vi "DRAM read write process.vi"(5 "debug ctr reset":bool, 6 "dram.reset":bool, 8 "dram mode":T3, 11 "DRAM resources":T1={"DRAM read data FIFO"="", "DRAM write data FIFO"="", "DRAM request FIFO"="", "DRAM U512 memo"=refnum, "DMA data loader"="custom data", "BRAM read data FIFO"="", "BRAM write data FIFO"="", "BRAM request FIFO"="", "BRAM U512 memo"=refnum}) -> (2 "DRAM debug ctr":T2, 3 "last written addr":u32)   [LabVIEW 2019, in "TX burst sequencer.lvlib"]
doc: "Handles writing and reading from DRAM.\nHas 3 interface FIFOs:\n- Write FIFO: provides data to write (addr + data)\n- Request FIFO: provides requests for data read\n- Read FIFO: takes data read from DRAM\n\nVI has 3 main states:\n- write (only write operations are executed with max throughput)\n- read (only read operations are executed with max throughput)\n- flush (empties Write and Request FIFO)"
uses:
  TX burst sequencer.lvlib
  DRAM mode.ctl
  DRAM resources.ctl
  <instrlib>/_niInstr/Memory/v1/FPGA/DRAM U512/niInstr Memory DRAM U512 v1 FPGA.lvclass
  <instrlib>/_niInstr/Memory/v1/FPGA/BRAM U512/niInstr Memory BRAM U512 v1 FPGA.lvclass
  <instrlib>/_niInstr/Memory/v1/FPGA/Memory/Public/Write Data (With Byte Enables).ctl
  <instrlib>/_niInstr/Memory/v1/FPGA/Memory/Public/Read Request.ctl
  <instrlib>/_niInstr/Memory/v1/FPGA/DRAM/Public/Timeslot Arbiter Configuration.ctl
  <vilib>/rvi/DataTransferAndStorage/Container/Common/niFpgaContainerExecOnDevCompGetState.vi
  <vilib>/rvi/Emulation/niFpgaEmulationIsFPGAContextNoSignature.vi
  <vilib>/rvi/Emulation/niFpgaSctlEmulationGetInTimedLoop.vi
  <vilib>/rvi/errors/niFpgaSetErrorForExecOnDevCompSimple.vi
  <vilib>/rvi/eio/common/nirviEmuReportErrorAndStop.vi
  <vilib>/rvi/DataTransferAndStorage/Container/Common/niFpgaContainerGetUniqueNameForEmu.vi
  <vilib>/rvi/FIFO/Fifo_Resource/nirvififoEmulationSetSize.vi
  <vilib>/rvi/FIFO/Fifo_Resource/nirviFifoEmulationQueueMgr.vi
  <instcachedir>/0/nirviFifoEmulationQueueMgr_E5CAEC123FF24DC58D834DCA3CDAA9B5.lvgen/nirviFifoEmulationQueueMgr_E5CAEC123FF24DC58D834DCA3CDAA9B5_017.vi
  <vilib>/rvi/FIFO/Fifo_Resource/nirvififoEmulationDetermineInputValidOut.vi
  <vilib>/rvi/FIFO/Fifo_Resource/nirvififoEmulationCreateLock.vi
  <vilib>/rvi/Emulation/niFpgaProcessEmulError.vi
  <vilib>/rvi/FIFO/Fifo_Resource/nirvififoEmulationObtainLock.vi
  <vilib>/rvi/FIFO/Fifo_Resource/nirvififoEmulationReleaseLock.vi
  <vilib>/rvi/occurrence/nirviWaitOnOccurrenceBase.vi
  <vilib>/rvi/errors/nirviReportUnexpectedCaseInternalError.vi
  <vilib>/rvi/errors/nirviReportUnexpectedCaseInternalError (U32).vi
  <vilib>/Utility/error.llb/Clear Errors.vi
  <vilib>/rvi/interface/RandomDataEmulation/niFpgaRandomDataHandleErrors.vi
  <instcachedir>/0/nirviFifoEmulationQueueMgr_E5CAEC123FF24DC58D834DCA3CDAA9B5.lvgen/nirviFifoEmulationQueueMgr_E5CAEC123FF24DC58D834DCA3CDAA9B5_003.vi
  <instrlib>/_niInstr/Basic Elements/v1/FPGA/Private/Count Up U32.vi
  <instcachedir>/0/nirviFifoEmulationQueueMgr_E5CAEC123FF24DC58D834DCA3CDAA9B5.lvgen/nirviFifoEmulationQueueMgr_E5CAEC123FF24DC58D834DCA3CDAA9B5_011.vi
  <vilib>/rvi/DataTransferAndStorage/Container/XNode/niFpgaContainer.xnode
  <vilib>/rvi/FIFO/Fifo_Resource/niFpgaFifoEmulationRefIn.vi
  <instrlib>/_niInstr/Memory/v1/FPGA/Memory/niInstr Memory v1 FPGA.lvclass
  <instrlib>/_niInstr/Memory/v1/FPGA/DRAM/niInstr Memory DRAM v1 FPGA.lvclass
  <instrlib>/_niInstr/Basic Elements/v1/FPGA/niInstr Basic Elements v1 FPGA.lvlib
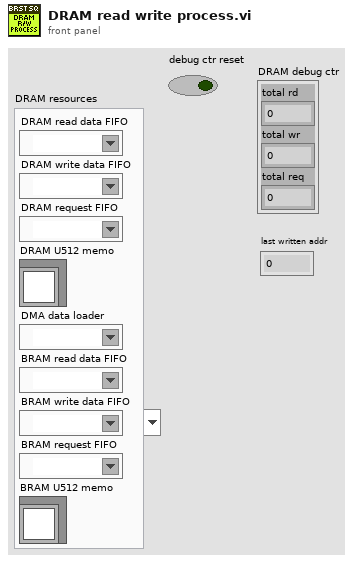
[diagram p1: front panel]
types:
  T1 = typedef "TX burst sequencer.lvlib/DRAM resources.ctl" = cluster{"DRAM read data FIFO":refnum<k21>, "DRAM write data FIFO":refnum<k21>, "DRAM request FIFO":refnum<k21>, "DRAM U512 memo":refnum<class "niInstr Memory DRAM U512 v1 FPGA.lvclass">, "DMA data loader":refnum<k21>, "BRAM read data FIFO":refnum<k21>, "BRAM write data FIFO":refnum<k21>, "BRAM request FIFO":refnum<k21>, "BRAM U512 memo":refnum<class "niInstr Memory BRAM U512 v1 FPGA.lvclass">}
  T2 = cluster{"total rd":u32, "total wr":u32, "total req":u32}
  T3 = typedef "TX burst sequencer.lvlib/DRAM mode.ctl" = enum16{"flush", "reset", "write", "read"}
  T4 = typedef "niInstr Memory v1 FPGA.lvclass/Read Request.ctl" = cluster{"address":u32, "valid":bool}
  T5 = typedef "niInstr Memory v1 FPGA.lvclass/Write Data (With Byte Enables).ctl" = cluster{"address":u32, "data":bool[], "byte enables":bool[], "valid":bool}
  T6 = typedef "niInstr Memory DRAM v1 FPGA.lvclass/Timeslot Arbiter Configuration.ctl" = cluster{"write grant time (clocks)":u16, "read grant time (clocks)":u16}
  T7 = typedef "niInstr Memory v1 FPGA.lvclass/Retrieve Data.ctl" = cluster{"data":bool[], "valid":bool}
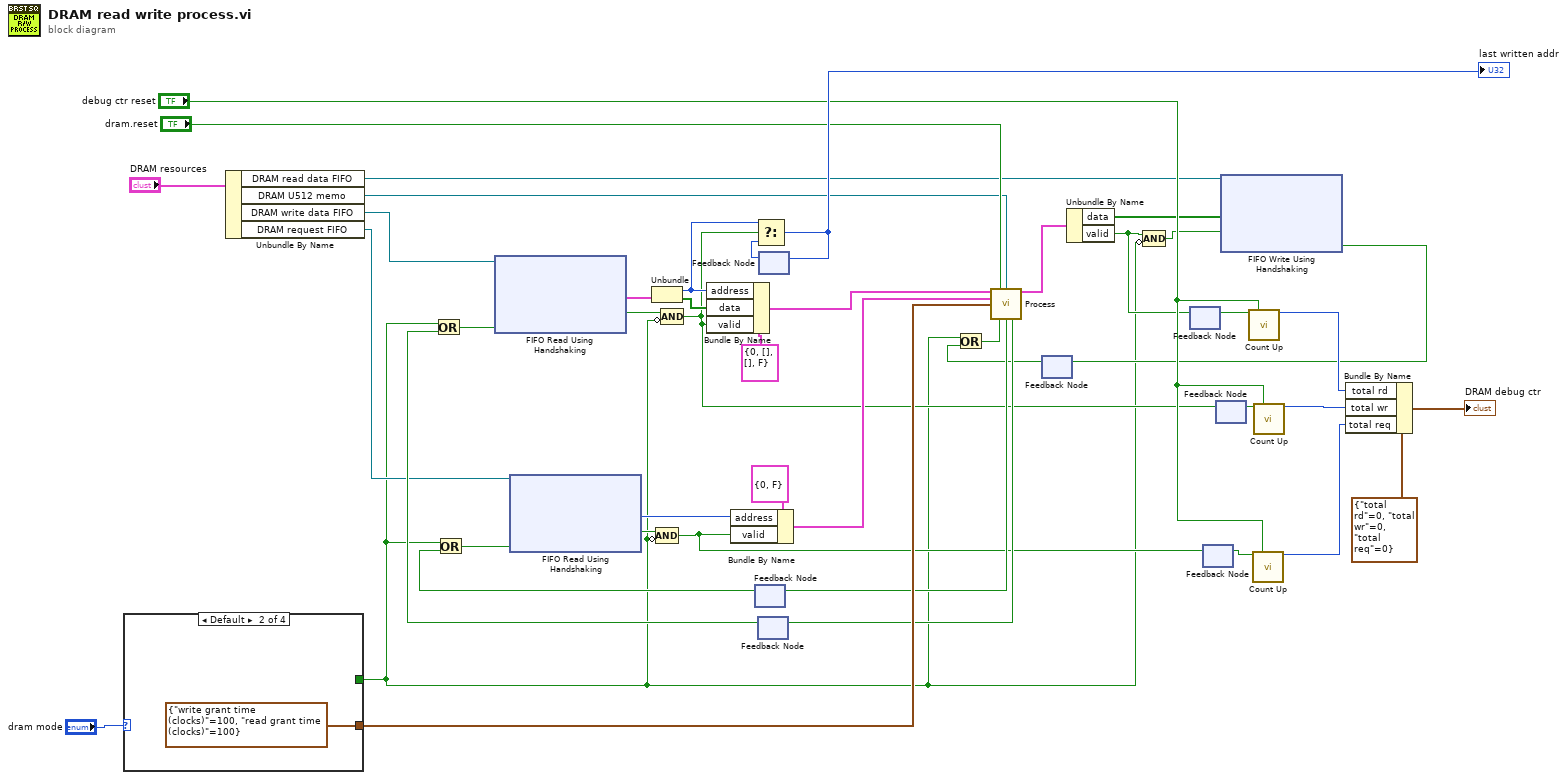
[diagram p0: block diagram]
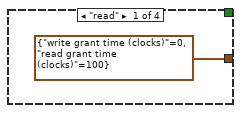
[diagram p2: hidden frame]
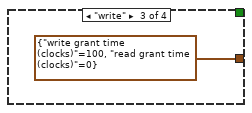
[diagram p3: hidden frame]
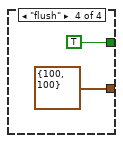
[diagram p4: hidden frame]
diagram:
  n1 = case shown="Default" "dram mode" {
    tunnel: [T6 {"write grant time (clocks)"=0, "read grant time (clocks)"=100} ("arbiter configuration") T6 {"write grant time (clocks)"=100, "read grant time (clocks)"=100} ("arbiter configuration") T6 {"write grant time (clocks)"=100, "read grant time (clocks)"=0} ("arbiter configuration") T6 {"write grant time (clocks)"=100, "read grant time (clocks)"=100} ("arbiter configuration")] -> w31
    tunnel: [_ _ _ TRUE] -> w2
    frame "read" {
    }
    frame Default {
    }
    frame "write" {
    }
    frame "flush" {
    }
  }
  n2 = Unbundle By Name("DRAM resources") -> ("DRAM read data FIFO"=w14:refnum<k21>, "DRAM U512 memo"=w13:refnum<class "niInstr Memory DRAM U512 v1 FPGA.lvclass">, "DRAM write data FIFO"=w12:refnum<k21>, "DRAM request FIFO"=w11:refnum<k21>)
  n3 = feedback #1() -> (w30:bool)  [unwired: 1 in]
  n4 = Or(x=w2, y=w30) -> (x .or. y?=w10:bool)
  n5 = xnode ("FIFO Read Using Handshaking")("Ready for Output"=w10, "FIFO In"=w11) -> ("Element"=w27:u32, "Output Valid"=w35:bool)  [unwired: 1 out]
  n6 = Compound Arithmetic op=AND(w35, invert w2) -> (w8:bool)
  n7 = Bundle By Name(cluster=T4 {"address"=0, "valid"=FALSE} ("request data"), "address"=w27, "valid"=w8) -> (w28:T4)
  n8 = feedback #2() -> (w21:bool)  [unwired: 1 in]
  n9 = Or(x=w2, y=w21) -> (x .or. y?=w9:bool)
  n10 = xnode ("FIFO Read Using Handshaking")("Ready for Output"=w9, "FIFO In"=w12) -> ("Element"=w22:cluster{"addr":u32, "data":bool[]}, "Output Valid"=w7:bool)  [unwired: 1 out]
  n11 = Unbundle(w22) -> ("addr"=w37:u32, "data"=w25:bool[])
  n12 = Compound Arithmetic op=AND(w7, invert w2) -> (w6:bool)
  n13 = Bundle By Name(cluster=T5 {"address"=0, "data"=[], "byte enables"=[], "valid"=FALSE} ("write"), "address"=w37, "data"=w25, "valid"=w6) -> (w24:T5)
  n14 = feedback #3() -> (w39:u32)  [unwired: 1 in]
  n15 = Select(t=w37, s=w6, f=w39) -> (s? t:f=w38:u32)
  "last written addr" <- w38
  n16 = feedback-in #3(w38) -> ()
  n17 = feedback #4() -> (w5:bool)  [unwired: 1 in]
  n18 = Or(x=w2, y=w5) -> (x .or. y?=w4:bool)
  n19 = call-dynamic "Process.vi"("write"=w24, "reset"="dram.reset", "memory"=w13, "request data"=w28, "arbiter configuration"=w31, "ready for retrieve data (T)"=w4) -> ("retrieve data"=w17:T7, "ready for request data"=w29:bool, "ready for write"=w20:bool)  [unwired: 6 in, 1 out]
  n20 = feedback-in #1(w29) -> ()
  n21 = feedback-in #2(w20) -> ()
  n22 = Unbundle By Name(w17) -> ("data"=w18:bool[], "valid"=w3:bool)
  n23 = Compound Arithmetic op=AND(w3, invert w2) -> (w1:bool)
  n24 = feedback #5() -> (w33:bool)  [unwired: 1 in]
  n25 = feedback-in #5(w3) -> ()
  n26 = feedback #6() -> (w34:bool)  [unwired: 1 in]
  n27 = feedback-in #6(w8) -> ()
  n28 = feedback #7() -> (w32:bool)  [unwired: 1 in]
  n29 = feedback-in #7(w6) -> ()
  n30 = xnode ("FIFO Write Using Handshaking")("Element"=w18, "Input Valid"=w1, "FIFO In"=w14) -> ("Ready for Input"=w19:bool)  [unwired: 1 out]
  n31 = feedback-in #4(w19) -> ()
  n32 = call-poly <instrlib>:"Count Up.vi"("increment"=w33, "reset"="debug ctr reset") -> ("count out"=w41:u32)  [unwired: 13 in]
  n33 = call-poly <instrlib>:"Count Up.vi"("increment"=w34, "reset"="debug ctr reset") -> ("count out"=w43:u32)  [unwired: 13 in]
  n34 = call-poly <instrlib>:"Count Up.vi"("increment"=w32, "reset"="debug ctr reset") -> ("count out"=w42:u32)  [unwired: 13 in]
  n35 = Bundle By Name(cluster=T2 {"total rd"=0, "total wr"=0, "total req"=0} ("input cluster"), "total rd"=w41, "total wr"=w42, "total req"=w43) -> (→"DRAM debug ctr":T2)
